vi "Update Menu Controls Highlight.vi"(8 "Error In":errorcluster, 9 "Selected Index":i32, 10 "Controls":refnum<vi>[](array[refnum]), 11 "State":enum16{"Init", "Update"}(ring)=enum."Update") -> (0 "Error Out":errorcluster)   [LabVIEW 2020, in "LMH-LINX.lvlib"]
uses:
  LMH-LINX.lvlib
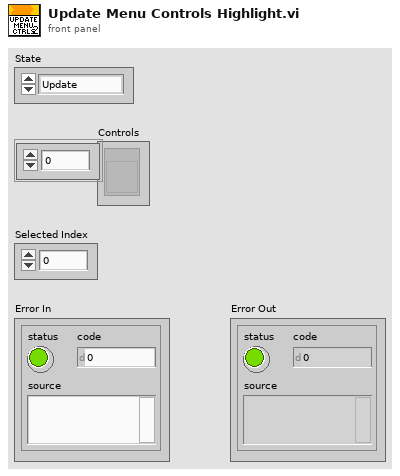
[diagram p1: front panel]
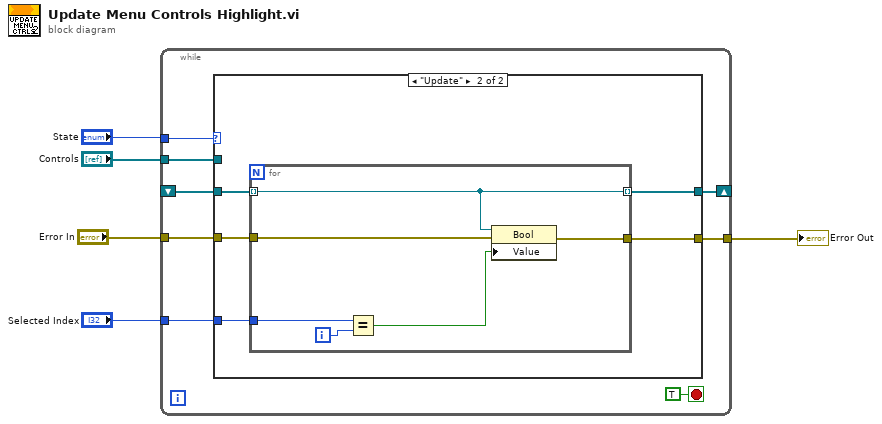
[diagram p0: block diagram]
diagram:
  n1 = while {
    tunnel: "Selected Index" -> [w13]
    shift-right: [w9] -> _
    shift-left: _ -> [w8]
    tunnel: "State" -> [w11]
    tunnel: "Controls" -> [w10]
    tunnel: [w7] -> w2
    tunnel: "Error In" -> [w6]
    stop <- TRUE stop-if-true
    n2 = case shown="\"Update\"" w11 {
      tunnel: w13 -> [_ w20]
      tunnel: [w15 w18] -> w9
      tunnel: w10 -> [w15 _]
      tunnel: w8 -> [_ w19]
      tunnel: [w14 w17] -> w7
      tunnel: w6 -> [w14 w16]
      frame "Init", Default {
      }
      frame "Update" {
        n3 = for {
          tunnel: w19 -> [w23] mode=indexing
          tunnel: w20 -> [w25]
          tunnel: [w24] -> w17
          tunnel: [w23] -> w18 mode=indexing
          tunnel: w16 -> [w22]
          i -> [w26]
          n4 = Equal?(x=w25, y=w26) -> (x = y?=w21:bool)
          n5 = property class="Bool"(reference=w23, error in=w22, "Value"=w21) -> (error out=w24:errorcluster)  [unwired: 1 out]
        }
      }
    }
  }
  "Error Out" <- w2
